vi "Auto 8.vi"(8 "Error In":errorcluster) -> (0 "Error Out":errorcluster)   [LabVIEW 2014]
uses:
  Global Variables/Refnum Names.vi
  <vilib>/Rock Robotics/Network Tables/SD Read Boolean.vi
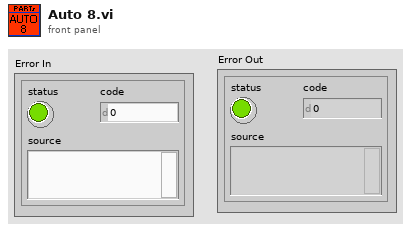
[diagram p1: front panel]
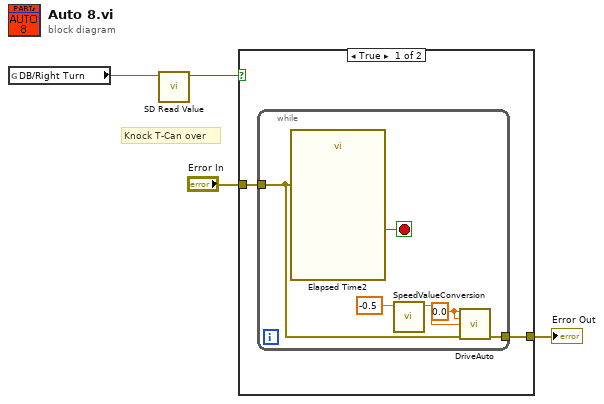
[diagram p0: block diagram]
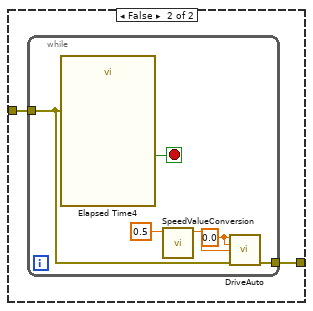
[diagram p2: hidden frame]
diagram:
  # "Knock T-Can over"
  n1 = global read "Refnum Names.vi" "DB/Right Turn"() -> (w1:string)
  n2 = call-poly <vilib>:"SD Read Value.vi"("Name"=w1) -> ("Boolean"=w4:bool)  [unwired: 8 in, 2 out]
  n3 = case shown="True" w4 {
    tunnel: "Error In" -> [w6 w14]
    tunnel: [w5 w13] -> w2
    frame True {
      n4 = while {
        tunnel: w6 -> [w9]
        tunnel: [w11] -> w5
        stop <- w10 stop-if-true
        w12 = 0.0 ("Arm Value")
        n5 = call "Elapsed Time2"("error in (no error)"=w9) -> ("Time has Elapsed"=w10:bool)  [unwired: 11 in, 7 out]
        n6 = call "SpeedValueConversion.vi"("Motor Value In"=-0.5 ("X In")) -> ("New to Old Conversion Value Out"=w7:dbl)  [unwired: 9 in, 1 out]
        n7 = call "DriveAuto.vi"("X In"=w12, "Y In"=w12, "R In"=w7, "Error In"=w9) -> ("Error Out"=w11:errorcluster)  [unwired: 11 in]
      }
    }
    frame False {
      n8 = while {
        tunnel: w14 -> [w17]
        tunnel: [w20] -> w13
        stop <- w18 stop-if-true
        w19 = 0.0 ("Arm Value")
        n9 = call "Elapsed Time4"("error in (no error)"=w17) -> ("Time has Elapsed"=w18:bool)  [unwired: 11 in, 7 out]
        n10 = call "SpeedValueConversion.vi"("Motor Value In"=0.5 ("X In")) -> ("New to Old Conversion Value Out"=w15:dbl)  [unwired: 9 in, 1 out]
        n11 = call "DriveAuto.vi"("X In"=w19, "Y In"=w19, "R In"=w15, "Error In"=w17) -> ("Error Out"=w20:errorcluster)  [unwired: 11 in]
      }
    }
  }
  "Error Out" <- w2
